vi "Send Launch Logger Msg.vi"(8 "error in (no error)":errorcluster, 9 "Log Level":T2, 10 "Logger Name":T1, 11 "Logger Mananger in":refnum<class "Logger Mananger.lvclass">) -> (0 "error out":errorcluster, 3 "Logger Mananger out":refnum<class "Logger Mananger.lvclass">)   [LabVIEW 2020, in "Logging.lvlib" / "Logger Mananger.lvclass"]
uses:
  Logger Mananger.lvclass
  C:/Program Files (x86)/National Instruments/LabVIEW 2020/vi.lib/ActorFramework/Actor/Actor.lvclass
  Define/Log Level.ctl
  Define/Log Option.ctl
  <vilib>/ActorFramework/Actor/Actor.lvclass/Actor.ctl
  <vilib>/ActorFramework/Message Enqueuer/Message Enqueuer.lvclass/Message Enqueuer.ctl
  Logger Mananger Messages/Luanch Logger Msg/Luanch Logger Msg.lvclass/Luanch Logger Msg.ctl
  <vilib>/ActorFramework/Message Enqueuer/Init from Existing Queue.vi
  <vilib>/ActorFramework/Message Enqueuer/Enqueue.vi
  Logger Mananger Messages/Luanch Logger Msg/Luanch Logger Msg.lvclass
  C:/Program Files (x86)/National Instruments/LabVIEW 2020/vi.lib/ActorFramework/Message/Message.lvclass
  <vilib>/ActorFramework/Message Priority Queue/Priority Enqueue.vi
  <vilib>/ActorFramework/Message Enqueuer/Message Enqueuer.lvclass
  <vilib>/ActorFramework/Actor/Actor.lvclass
  Logging.lvlib
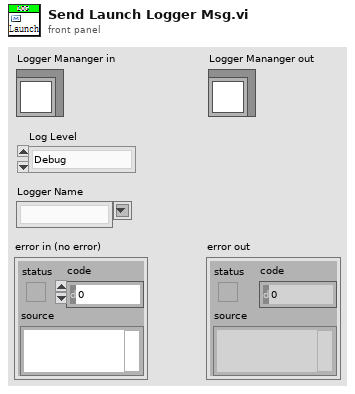
[diagram p1: front panel]
types:
  T1 = typedef "Logging.lvlib/Log Option.ctl" = string
  T2 = typedef "Logging.lvlib/Log Level.ctl" = enum16{"Debug", "Info", "Warn", "Error"}
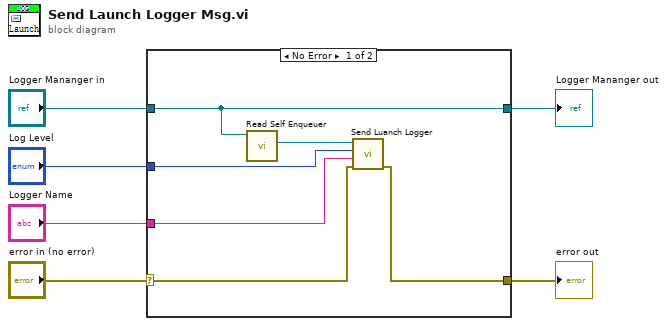
[diagram p0: block diagram]
diagram:
  n1 = case shown="No Error" "error in (no error)" {
    selector: "error in (no error)" -> [w8 w14]
    tunnel: [w7 w14] -> w5
    tunnel: [w12 w13] -> w3
    tunnel: "Logger Mananger in" -> [w12 w13]
    tunnel: "Logger Name" -> [w10 _]
    tunnel: "Log Level" -> [w9 _]
    frame No Error {
      n2 = call <vilib>:"Read Self Enqueuer.vi"("Actor"=w12) -> ("Self Enqueuer"=w11:refnum<class "Message Enqueuer.lvclass">)  [unwired: 10 in]
      n3 = call "Send Luanch Logger.vi"("error in (no error)"=w8, "Class Name"=w10, "Log Level"=w9, "Message Enqueuer"=w11) -> ("error out"=w7:errorcluster)  [unwired: 6 in, 1 out]
    }
    frame Error {
    }
  }
  "error out" <- w5
  "Logger Mananger out" <- w3
